vi "RPC Method TestDataTypes.vi"(8 "error in (no error)":errorcluster, 11 "OOP Server in":refnum<class "Data Marshal Server.lvclass">) -> (0 "error out":errorcluster, 3 "OOP Server out":refnum<class "Data Marshal Server.lvclass">)   [LabVIEW 2019, in "Data Marshal Server.lvlib" / "Data Marshal Server.lvclass"]
uses:
  Data Marshal Server.lvclass
  RPC Messages/TestDataTypesParameters/TestDataTypesParameters_Data.ctl
  RPC Messages/DataTypeTest/DataTypeTest_Data.ctl
  Data Marshal Server.lvclass/Data Marshal Server.ctl
panel:
  out "Data":string
  out "Message Data":T1
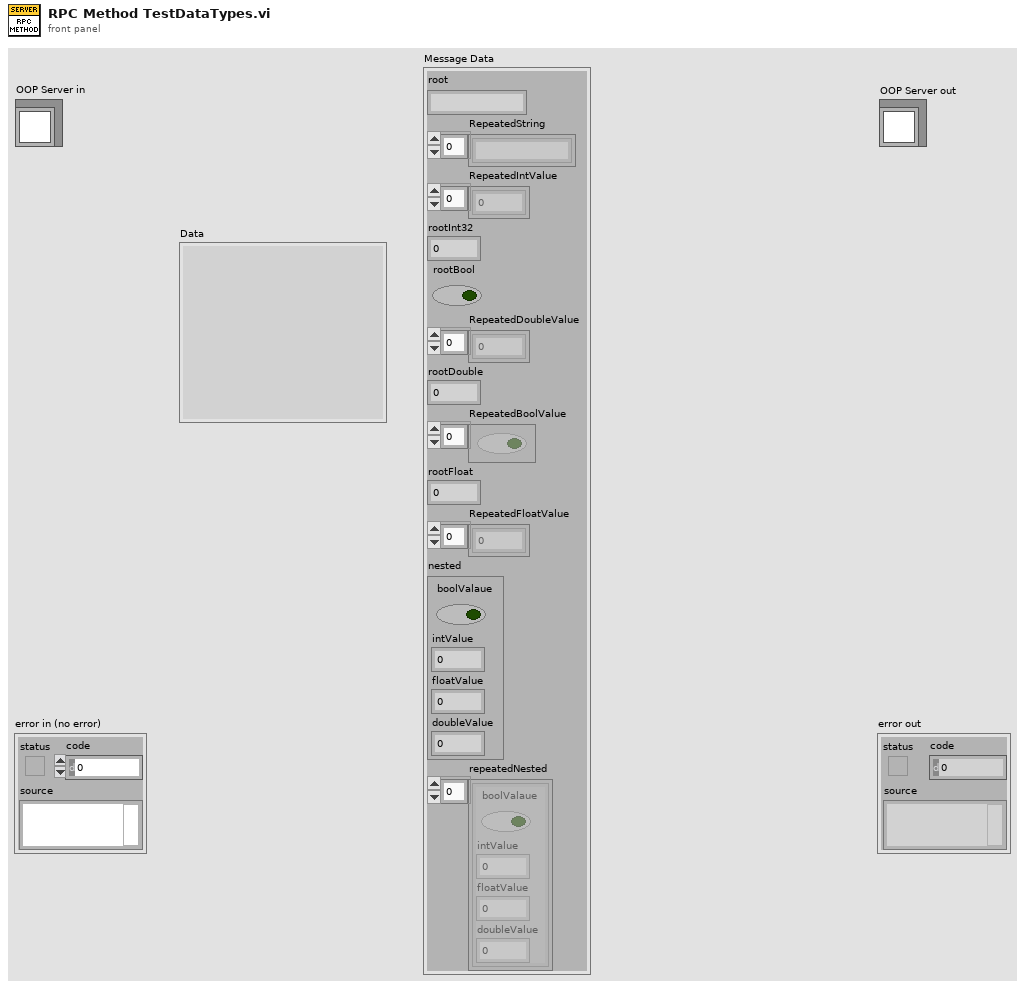
[diagram p1: front panel]
types:
  T1 = typedef "Data Marshal Server.lvlib/Data Marshal Server.lvclass/TestDataTypesParameters_Data.ctl" = cluster{"root":string, "RepeatedString":string[], "RepeatedIntValue":i32[], "rootInt32":i32, "rootBool":bool, "RepeatedDoubleValue":dbl[], "rootDouble":dbl, "RepeatedBoolValue":bool[], "rootFloat":sgl, "RepeatedFloatValue":sgl[], "nested":T2, "repeatedNested":T2[]}
  T2 = typedef "Data Marshal Server.lvlib/Data Marshal Server.lvclass/DataTypeTest_Data.ctl" = cluster{"boolValaue":bool, "intValue":i32, "floatValue":sgl, "doubleValue":dbl}
  T3 = typedef "Data Marshal Server.lvlib/Data Marshal Server.lvclass/Server Internal UEs.ctl" = cluster{"Invoke Internal UE":refnum<user-event>, "Query Internal UE":refnum<user-event>, "Register Internal UE":refnum<user-event>, "TestDataTypes Internal UE":refnum<user-event>}
  T4 = typedef "Data Marshal Server.lvlib/Data Marshal Server.lvclass/Server gRPC UEs.ctl" = cluster{"Invoke gRPC UE":refnum<user-event>, "Query gRPC UE":refnum<user-event>, "Register gRPC UE":refnum<user-event>, "TestDataTypes gRPC UE":refnum<user-event>}
  T5 = typedef "Data Marshal Server.lvlib/gprc-lvsupport.lvlib/grpcId.ctl" = u64
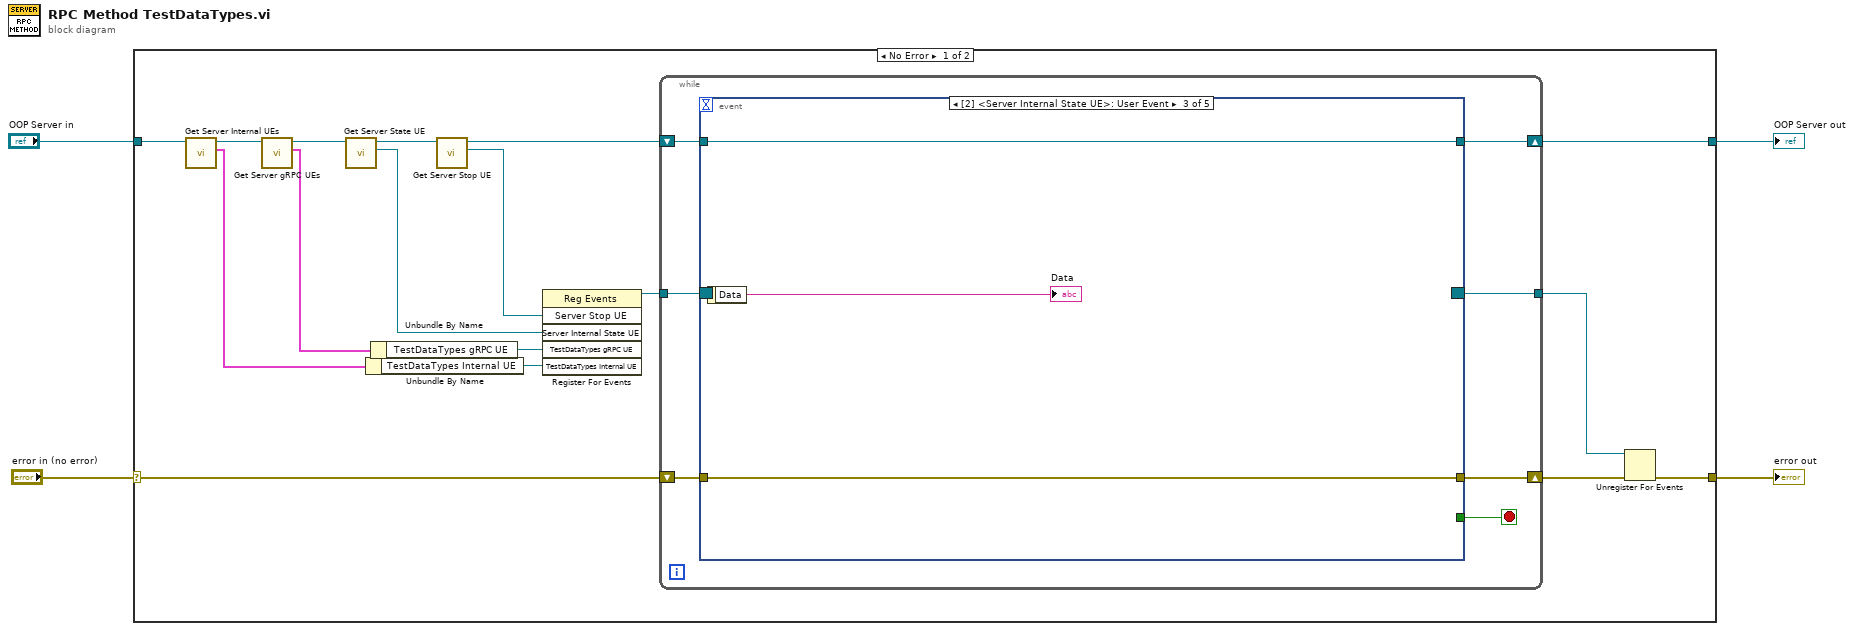
[diagram p0: block diagram]
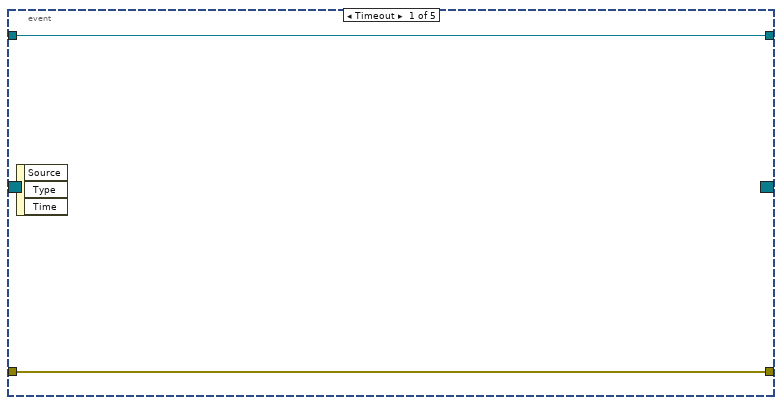
[diagram p2: hidden frame]
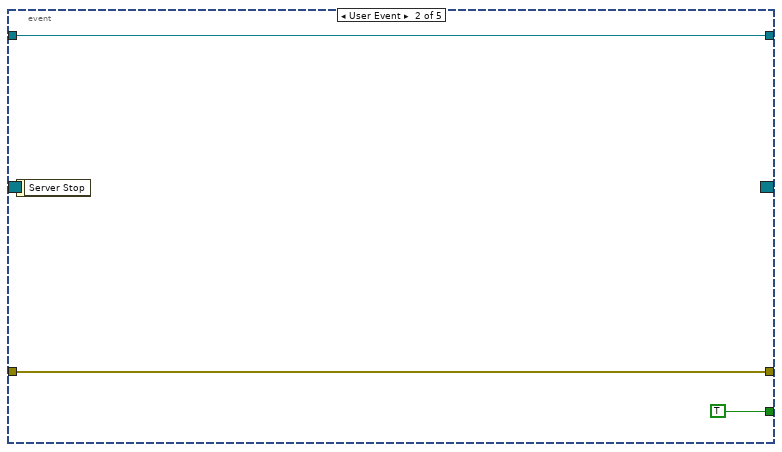
[diagram p3: hidden frame]
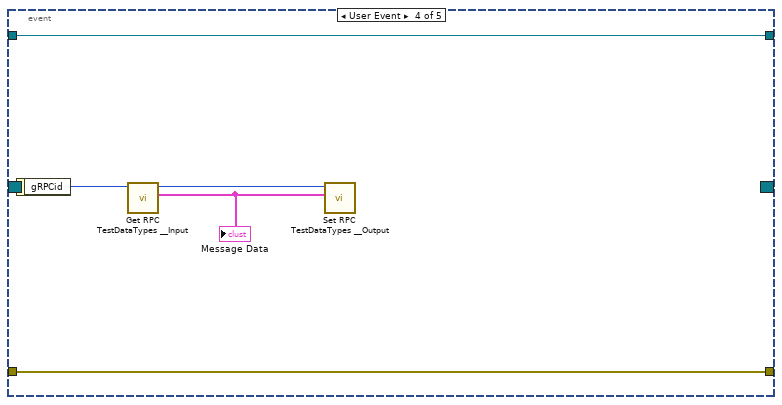
[diagram p4: hidden frame]
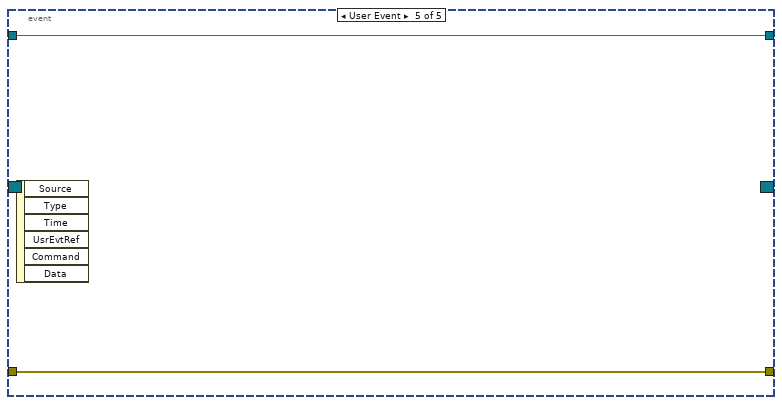
[diagram p5: hidden frame]
diagram:
  n1 = case shown="No Error" "error in (no error)" {
    selector: "error in (no error)" -> [w17 w45]
    tunnel: [w15 w45] -> w3
    tunnel: "OOP Server in" -> [w19 w44]
    tunnel: [w5 w44] -> w1
    frame No Error {
      n2 = call "Get Server Internal UEs.vi"("OOP Server in"=w19) -> ("Server Internal UEs"=w11:T3, "OOP Server out"=w18:refnum<class "Data Marshal Server.lvclass">)  [unwired: 9 in]
      n3 = call "Get Server gRPC UEs.vi"("OOP Server in"=w18) -> ("Server gRPC UEs"=w13:T4, "OOP Server out"=w8:refnum<class "Data Marshal Server.lvclass">)  [unwired: 9 in]
      n4 = call "Get Server State UE.vi"("Template Server in"=w8) -> ("Server Internal State UE"=w6:refnum<user-event>, "Template Server out"=w7:refnum<class "Data Marshal Server.lvclass">)  [unwired: 9 in]
      n5 = Unbundle By Name ("Unbundle Internal UE")(w11) -> ("TestDataTypes Internal UE"=w10:refnum<user-event>)
      n6 = Unbundle By Name ("Unbundle gRPC UE")(w13) -> ("TestDataTypes gRPC UE"=w12:refnum<user-event>)
      n7 = call "Get Server Stop UE.vi"("OOP Server in"=w7) -> ("Server Stop UE"=w21:refnum<user-event>, "OOP Server out"=w9:refnum<class "Data Marshal Server.lvclass">)  [unwired: 9 in]
      n8 = register-events(w21, w6, w12, w10) -> (reference out=w20:refnum<event-registration>)  [unwired: 2 in, 1 out]
      n9 = while {
        tunnel: w20 -> [w28]
        tunnel: [w24] -> w14
        shift-right: [w25] -> w16
        shift-left: w17 -> [w26]
        shift-right: [w22] -> w5
        shift-left: w9 -> [w23]
        stop <- w27 stop-if-true
        n10 = event "RPC Method Event Structure" shown="[2] <Server Internal State UE>: User Event" {
          selector: w28 -> [_ _ _ _ _]
          dyn-events: [_ _ _ _ _] -> w24
          timeout: _ -> [_ _ _ _ _]
          tunnel: [_ TRUE _ _ _] -> w27
          tunnel: w26 -> [w30 w32 w36 w41 w43]
          tunnel: [w30 w32 w36 w41 w43] -> w25
          tunnel: w23 -> [w29 w31 w35 w40 w42]
          tunnel: [w29 w31 w35 w40 w42] -> w22
          event Timeout {
            n11 = event-data() -> ()  [unwired: 1 in, 3 out]
          }
          event User Event {
            n12 = event-data() -> ()  [unwired: 1 in, 1 out]
          }
          event User Event {
            n13 = event-data() -> ("Data"=→"Data":string)  [unwired: 1 in]
          }
          event User Event {
            n14 = event-data() -> ("gRPCid"=w39:T5)  [unwired: 1 in]
            n15 = call "Get RPC TestDataTypes __Input.vi"("gRPCid in"=w39) -> ("Message Data"=w37:T1, "gRPCid out"=w38:T5)  [unwired: 8 in, 1 out]
            "Message Data" <- w37
            n16 = call "Set RPC TestDataTypes __Output.vi"("Message Data"=w37, "gRPCid in"=w38) -> ()  [unwired: 9 in, 1 out]
          }
          event User Event {
            n17 = event-data() -> ()  [unwired: 1 in, 6 out]
          }
        }
      }
      n18 = Unregister For Events(event registration refnum=w14, error in=w16) -> (error out=w15:errorcluster)
    }
    frame Error {
    }
  }
  "error out" <- w3
  "OOP Server out" <- w1
